vi "Read Binary recovery File.vi"() -> (0 "error out":errorcluster, 3 "Data Out":dbl[](array[numeric]))   [LabVIEW 2020]
panel:
  in  "Path":path
  in  "error in (no error)":errorcluster
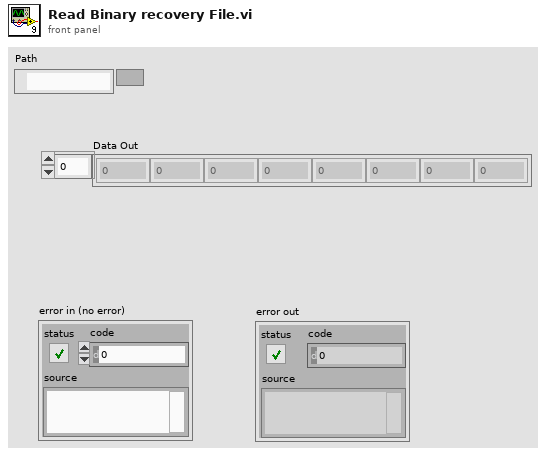
[diagram p1: front panel]
types:
  T1 = enum16{"open", "replace", "create", "open or create", "replace or create", "replace or create with confirmation"}
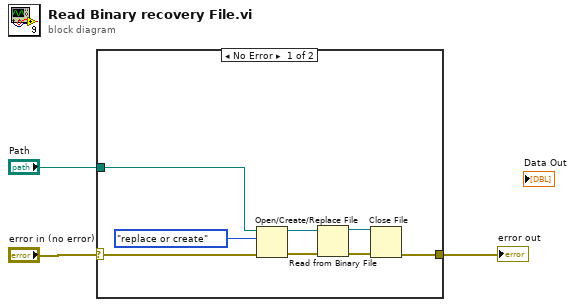
[diagram p0: block diagram]
diagram:
  n1 = case shown="No Error" "error in (no error)" {
    selector: "error in (no error)" -> [w10 w12]
    tunnel: "Path" -> [w11 _]
    tunnel: [w9 w12] -> w1
    frame No Error {
      n2 = Open/Create/Replace File(file path (use dialog)=w11, error in=w10, operation (0:open)=T1."replace or create") -> (refnum out=w4:refnum<file>, error out=w5:errorcluster)  [unwired: 3 in, 1 out]
      n3 = Read from Binary File(8:w5, 11:w4) -> (0:w6:errorcluster, 3:w7:refnum<file>)  [unwired: 4 in, 2 out]
      n4 = Close File(refnum=w7, error in=w6) -> (error out=w9:errorcluster)  [unwired: 1 out]
    }
    frame Error {
    }
  }
  "error out" <- w1
